vi "I_Sense_20kHz_v2.vi"(8 "error in":errorcluster) -> (0 "error out":errorcluster, 3 "Result":dbl[](array[numeric]))   [LabVIEW 2022 SP3]
uses:
  <vilib>/DAQmx/write.llb/DAQmx Write (Analog 1D Wfm NChan NSamp).vi
  <vilib>/DAQmx/read.llb/DAQmx Read (Analog 1D Wfm NChan NSamp).vi
  <vilib>/DAQmx/write.llb/DAQmx Write (Analog DBL 1Chan 1Samp).vi
  <vilib>/DAQmx/create/channels.llb/DAQmx Create Channel (AO-Voltage-Basic).vi
  <vilib>/DAQmx/configure/timing.llb/DAQmx Timing (Sample Clock).vi
  <vilib>/measure/mascope.llb/Amplitude and Levels N chan.vi
  <vilib>/DAQmx/miscellaneous.llb/DAQmx Fill In Error Info.vi
  <vilib>/measure/madcrms.llb/Basic Averaged DC-RMS for N Chan.vi
  <resource>/objmgr/daqmx.rc
  <vilib>/measure/NI_MABase.lvlib
  <vilib>/measure/NI_MAPro.lvlib
panel:
  out "DC Out":dbl[](array[numeric]) format="%.2p"
  out "Gains":dbl[](array[numeric])
  out "Amplitude Out":dbl[](array[numeric]) format="%.2p"
  out "High Out":dbl[](array[numeric]) format="%.2p"
  out "Low Out":dbl[](array[numeric]) format="%.2p"
  out "Amplitude In":dbl[](array[numeric]) format="%.2p"
  out "Low In":dbl[](array[numeric]) format="%.2p"
  out "High In":dbl[](array[numeric]) format="%.2p"
  in  "Sample Mode":i32(ring)=10123 items=["Finite Samples"=10178, "Continuous Samples"=10123, "Hardware Timed Single Point"=12522]
  out "Output Waveform":waveform(dbl)[](graph)=[{"t0"=timestamp(0 s since 1904-01-01), "dt"=0.001, "Y"=[]}]
  out "Input Waveform":waveform(dbl)[](graph)=[{"t0"=timestamp(0 s since 1904-01-01), "dt"=0.001, "Y"=[]}]
  in  "Number of Samples":i32=30
  in  "Sample Rate":dbl=300000.0
  in  "Sample Clock Source":tag="OnboardClock"
  out "Actual Sample Rate":dbl=1000.0 format="%0.2f"
  # "ISENSE_C+"
  # "ISENSE_C-"
  # "ISENSE_C+"
  # "ISENSE_C-"
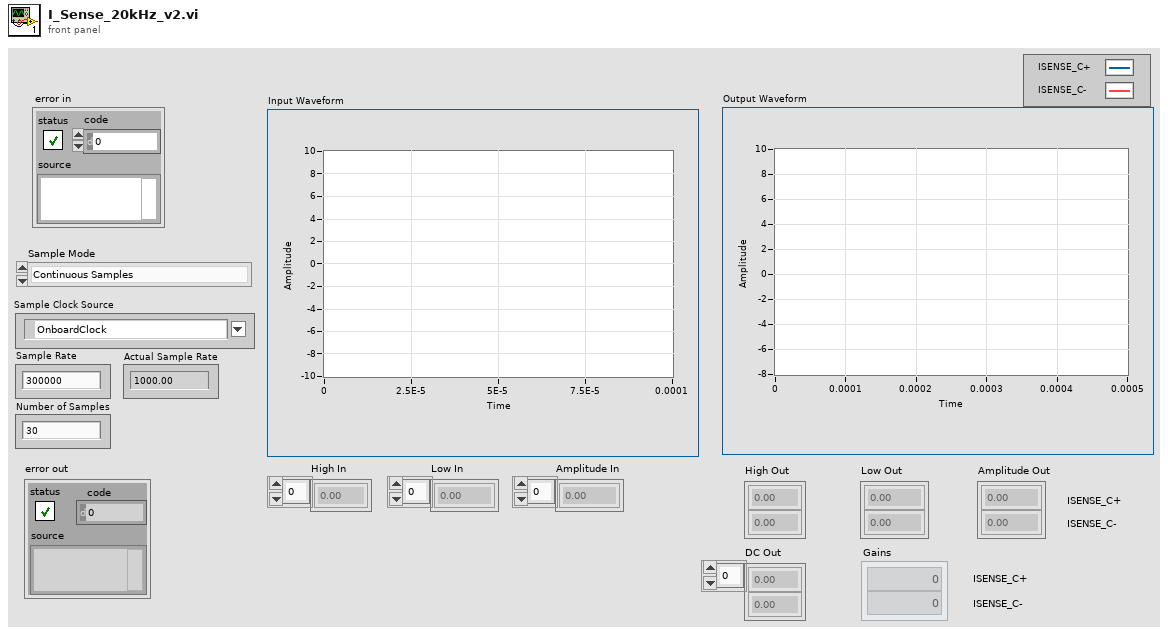
[diagram p1: front panel]
types:
  T1 = cluster{"Waveform Type":u16, "Amplitude":dbl, "Frequency":dbl}[]
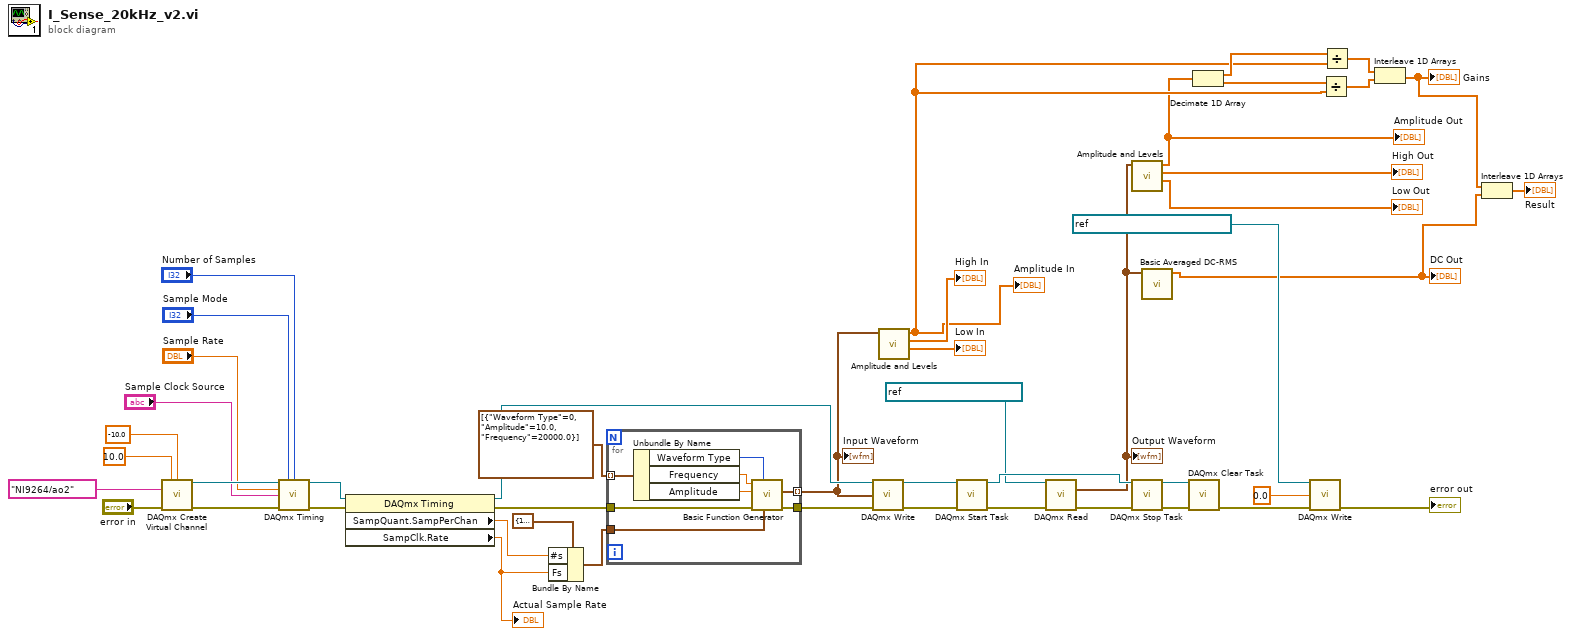
[diagram p0: block diagram]
diagram:
  n1 = call-poly <vilib>:"DAQmx Create Virtual Channel.vi"("maximum value"=10.0, "minimum value"=-10.0, "physical channels"=tag "NI9264/ao2", "error in"="error in") -> ("task out"=w43:refnum<k21>, "error out"=w44:errorcluster)  [unwired: 10 in]
  n2 = call-poly <vilib>:"DAQmx Timing.vi"("task/channels in"=w43, "sample mode"="Sample Mode", "samples per channel"="Number of Samples", "rate"="Sample Rate", "source"="Sample Clock Source", "error in"=w44) -> ("task out"=w47:refnum<k21>, "error out"=w46:errorcluster)  [unwired: 8 in]
  n3 = property class="DAQmx Timing"(reference=w47, error in=w46) -> (reference out=w27:refnum<k21>, error out=w28:errorcluster, "SampQuant.SampPerChan"=w33:dbl, "SampClk.Rate"=w32:dbl)
  "Actual Sample Rate" <- w32
  n4 = Bundle By Name(cluster=cluster{"Fs":dbl, "#s":dbl} {"Fs"=1000.0, "#s"=1000.0} ("sampling info"), "#s"=w33, "Fs"=w32) -> (w39:cluster{"Fs":dbl, "#s":dbl})
  n5 = for {
    tunnel: w28 -> [w55]
    tunnel: w39 -> [w54]
    tunnel: [w53] -> w36
    tunnel: T1 [{"Waveform Type"=0, "Amplitude"=10.0, "Frequency"=20000.0}] ("Output Array") -> [w52] mode=indexing
    tunnel: [w48] -> w20 mode=indexing
    n6 = Unbundle By Name(w52) -> ("Waveform Type"=w51:u16, "Frequency"=w50:dbl, "Amplitude"=w49:dbl)
    n7 = call <vilib>:"Basic Function Generator.vi"("sampling info"=w54, "signal type"=w51, "error in (no error)"=w55, "amplitude"=w49, "frequency"=w50) -> ("error out"=w53:errorcluster, "signal out"=w48:waveform(dbl))  [unwired: 4 in, 1 out]
  }
  "Input Waveform" <- w20
  n8 = call-poly <vilib>:"DAQmx Write.vi"("task/channels in"=w27, "data"=w20, "error in"=w36) -> ("task out"=w38:refnum<k21>, "error out"=w37:errorcluster)  [unwired: 10 in, 1 out]
  n9 = call-poly <vilib>:"Amplitude and Levels.vi"("signal(s) in"=w20) -> ("low state level"=→"Low In":dbl[], "high state level"=→"High In":dbl[], "amplitude"=w7:dbl[])  [unwired: 7 in, 1 out]
  "Amplitude In" <- w7
  n10 = call <vilib>:"DAQmx Start Task.vi"("task/channels in"=w38, "error in"=w37) -> ("task out"=w29:refnum<k21>, "error out"=w26:errorcluster)  [unwired: 12 in]
  n11 = call-poly <vilib>:"DAQmx Read.vi"("task/channels in"=refnum<k21> "BONTS_ISENSE_FAST", "error in"=w26) -> ("data"=w4:waveform(dbl)[], "error out"=w25:errorcluster)  [unwired: 11 in, 1 out]
  "Output Waveform" <- w4
  n12 = call-poly <vilib>:"Amplitude and Levels.vi"("signal(s) in"=w4) -> ("low state level"=→"Low Out":dbl[], "high state level"=→"High Out":dbl[], "amplitude"=w6:dbl[])  [unwired: 7 in, 1 out]
  "Amplitude Out" <- w6
  n13 = call <vilib>:"DAQmx Stop Task.vi"("task/channels in"=w29, "error in"=w25) -> ("task out"=w31:refnum<k21>, "error out"=w30:errorcluster)  [unwired: 12 in]
  n14 = call-poly <vilib>:"Basic Averaged DC-RMS.vi"("signals in"=w4) -> ("DC values"=w1:dbl[])  [unwired: 7 in, 3 out]
  "DC Out" <- w1
  n15 = call <vilib>:"DAQmx Clear Task.vi"("task in"=w31, "error in"=w30) -> ("error out"=w16:errorcluster)  [unwired: 13 in]
  n16 = Decimate 1D Array(w6) -> (w11:dbl[], w10:dbl[])
  n17 = call-poly <vilib>:"DAQmx Write.vi"("task/channels in"=refnum<k21> "BONTS_CurrentOutput_0", "data"=0.0, "error in"=w16) -> ("error out"=→"error out":errorcluster)  [unwired: 10 in, 2 out]
  n18 = Divide(x=w10, y=w7) -> (x/y=w8:dbl[])
  n19 = Divide(x=w11, y=w7) -> (x/y=w9:dbl[])
  n20 = Interleave 1D Arrays(w9, w8) -> (w2:dbl[])
  "Gains" <- w2
  n21 = Interleave 1D Arrays(w2, w1) -> (→"Result":dbl[])
